vi "State Control.vi"(10 "State":T1(ring)=enum."Pre-Primary", 11 "Action":enum16{"Get", "Set"}(ring)) -> (2 "State Out":T1(ring)=enum."Pre-Primary")   [LabVIEW 2013]
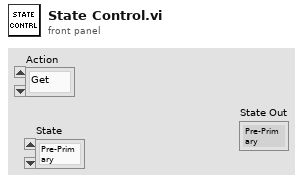
[diagram p1: front panel]
types:
  T1 = enum16{"Stopped", "Primary", "Secondary", "Pre-Primary"}
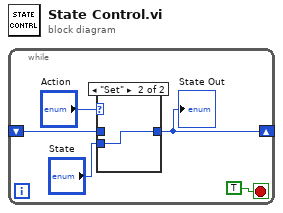
[diagram p0: block diagram]
diagram:
  n1 = while {
    shift-right: [w1] -> _
    shift-left: _ -> [w2]
    stop <- TRUE stop-if-true
    n2 = case shown="\"Set\"" "Action" {
      tunnel: [w6 w7] -> w1
      tunnel: "State" -> [_ w7]
      tunnel: w2 -> [w6 _]
      frame "Get", Default {
      }
      frame "Set" {
      }
    }
    "State Out" <- w1
  }
